vi "-8780 ReadRate not set--error.vi"(8 "error in":errorcluster) -> (0 "error out":errorcluster)   [LabVIEW 2024, in "Thermometer Multichannel Worker.lvlib" / "Thermometer Multichannel Worker.lvclass"]
uses:
  Thermometer Multichannel Worker.lvclass
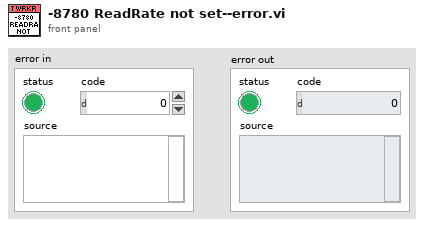
[diagram p1: front panel]
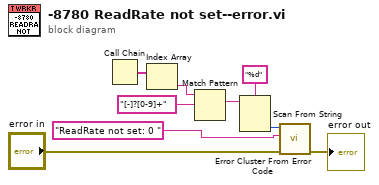
[diagram p0: block diagram]
diagram:
  n1 = Call Chain() -> (call chain=w7:string[])
  n2 = Index Array(array=w7) -> (element=w5:string)  [unwired: 1 in]
  n3 = Match Pattern(string=w5, regular expression="[-]?[0-9]+") -> (match substring=w4:string)  [unwired: 1 in, 3 out]
  n4 = Scan From String(format string="%d", input string=w4) -> (output 1=w2:i32)  [unwired: 3 in, 3 out]
  n5 = call <vilib>:"Error Cluster From Error Code.vi"("error in (no error)"="error in", "error message (\"\")"="ReadRate not set: 0 " ("error message (\"\")"), "error code (0)"=w2) -> ("error out"=→"error out":errorcluster)  [unwired: 6 in]
